vi "4CHDAQ - Configure Analog Output.vi"(6 "Cycles per Buffer":i32=5, 7 "Channel Name":string, 8 "Amplitude":dbl=1.0 format="%0.2p", 9 "Desired Frequency":dbl=1000.0 format="%.2f", 10 "Waveform Type":T1(ring), 11 "Physical Channels":tag="Dev1/ao0:1") -> (0 "error out":errorcluster, 2 "Resulting Frequency":dbl=1000.0 format="%.2f", 3 "task out":refnum<k21>)   [LabVIEW 2015]
uses:
  <vilib>/DAQmx/write.llb/DAQmx Write (Analog 1D Wfm NChan NSamp).vi
  <vilib>/DAQmx/create/channels.llb/DAQmx Create Channel (AO-Voltage-Basic).vi
  <vilib>/DAQmx/configure/timing.llb/DAQmx Timing (Use Waveform).vi
  <vilib>/DAQmx/miscellaneous.llb/DAQmx Fill In Error Info.vi
panel:
  in  "Samples per Buffer":dbl=250.0
  in  "Minimum Value":dbl=-10.0 format="%0.2f"
  in  "Maximum Value":dbl=10.0 format="%0.2f"
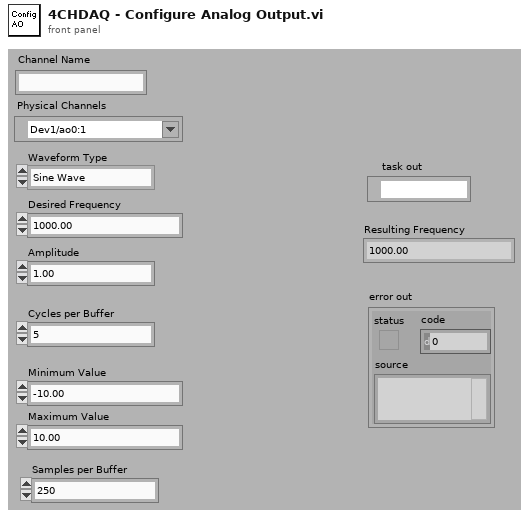
[diagram p1: front panel]
types:
  T1 = enum16{"Sine Wave", "Triangle Wave", "Square Wave", "Sawtooth Wave"}
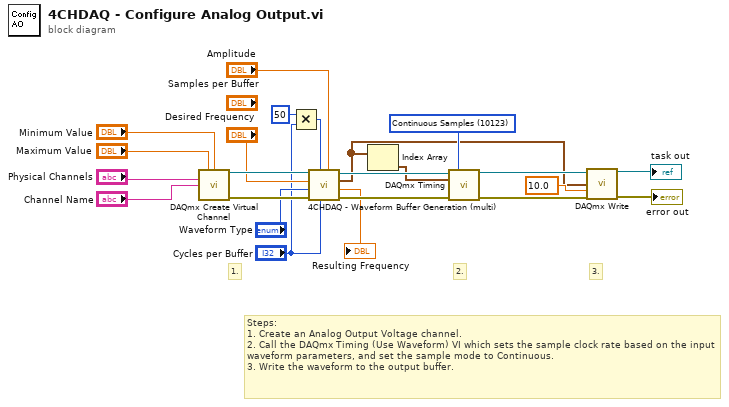
[diagram p0: block diagram]
diagram:
  w23 = 10123 items=["Finite Samples"=10178, "Continuous Samples"=10123] ("sample mode")
  # "Steps: \n1. Create an Analog Output Voltage channel.\n2. Call the DAQmx Timing (Use Waveform) VI which sets the sample clock rate based on the input waveform parameters, and set the sample mode to Continuous.\n3. Write the waveform to the output buffer."
  # "3."
  # "2."
  # "1."
  n1 = call-poly <vilib>:"DAQmx Create Virtual Channel.vi"("maximum value"="Maximum Value", "minimum value"="Minimum Value", "physical channels"="Physical Channels", "name to assign"="Channel Name") -> ("task out"=w14:refnum<k21>, "error out"=w13:errorcluster)  [unwired: 10 in]
  n2 = Multiply(x=50, y="Cycles per Buffer") -> (x*y=w3:i32)
  n3 = call "4CHDAQ - Waveform Buffer Generation (multi).vi"("Amplitude"="Amplitude", "Cycles per Buffer"="Cycles per Buffer", "Samples per Buffer"=w3, "error in (no error)"=w13, "Waveform Type"="Waveform Type", "Desired Frequency"="Desired Frequency", "task/channels in"=w14) -> ("error out"=w15:errorcluster, "Resulting Frequency"=→"Resulting Frequency":dbl, "Waveform"=w1:waveform(dbl)[], "task out"=w16:refnum<k21>)  [unwired: 1 out]
  n4 = Index Array(array=w1) -> (element=w9:waveform(dbl))  [unwired: 1 in]
  n5 = call-poly <vilib>:"DAQmx Timing.vi"("task/channels in"=w16, "sample mode"=w23, "waveform"=w9, "error in"=w15) -> ("task out"=w18:refnum<k21>, "error out"=w17:errorcluster)  [unwired: 10 in]
  n6 = call-poly <vilib>:"DAQmx Write.vi"("task/channels in"=w18, "data"=w1, "timeout"=10.0 ("Wirite Timeout"), "error in"=w17) -> ("task out"=→"task out":refnum<k21>, "error out"=→"error out":errorcluster)  [unwired: 9 in, 1 out]
